vi "STM_Server.vi"() -> ()   [LabVIEW 2019, in "RemoteControl.STM.lvclass"]
uses:
  RemoteControl.STM.lvclass
  <vilib>/NI/STM/SubVIs/MetaDataElement.ctl
  <vilib>/NI/STM/TCP/Write Meta Data (TCP Ref).vi
  <vilib>/NI/STM/TCP/Get Connection Reference (TCP).vi
  <vilib>/NI/STM/TCP/Write Meta Data (TCP Clst).vi
  <vilib>/NI/STM/TCP/Read Message (TCP).vi
  <vilib>/NI/STM/TCP/Write Message (TCP).vi
  <vilib>/NI/STM/NI STM.lvlib
panel:
  out "counter 2":u32
  out "counter":u32
  in  "service name":string
  out "remote address":string
  out "command received":T1
  in  "Enum":T2(ring)
  out "data received":string
  in  "stop":bool
  out "error out":errorcluster
  # "SERVER  (INSTRUMENT)"
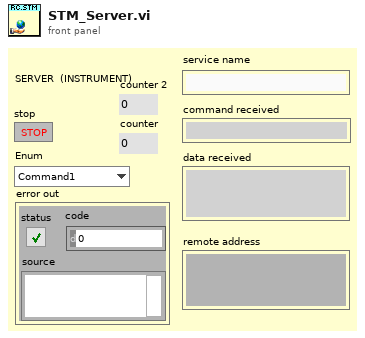
[diagram p1: front panel]
types:
  T1 = typedef "NI STM.lvlib/MetaDataElement.ctl" = string
  T2 = enum16{"Command1", "Command2", "Command3", "Command4", "HELP", "ACK", "CLOSE"}
  T3 = typedef "NI STM.lvlib/TCP Connection Info.ctl" = cluster{"connection ID":refnum<k5>, "meta data":T1[]}
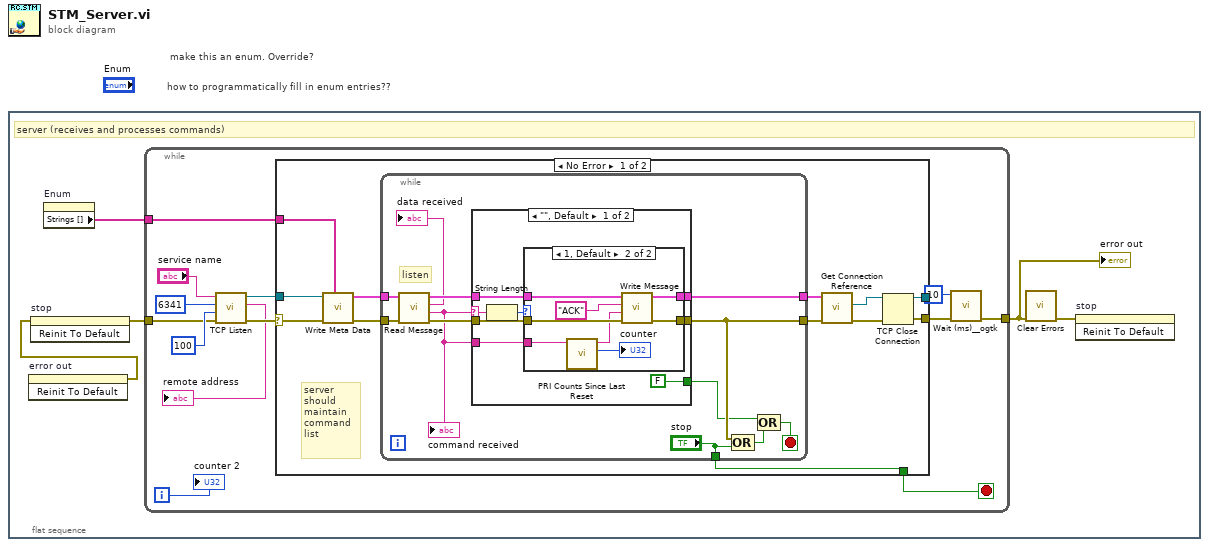
[diagram p0: block diagram]
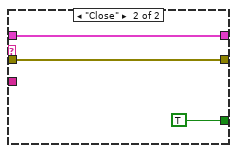
[diagram p3: hidden frame]
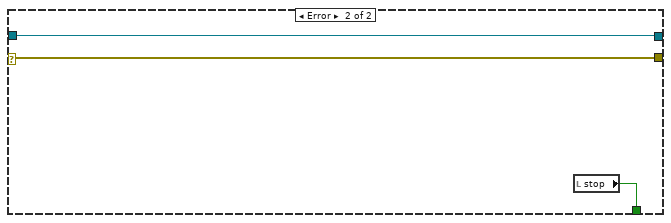
[diagram p4: hidden frame]
diagram:
  # "how to programmatically fill in enum entries??"
  # "make this an enum. Override?"
  n1 = flat-sequence {
    frame #0 {
      # "server (receives and processes commands)"
      n2 = invoke on="error out" class="Clust (strict)" method="Reinit To Default"() -> (error out=w1:errorcluster)  [unwired: 3 in, 2 out]
      n3 = invoke on="stop" class="Bool (strict)" method="Reinit To Default"(error in=w1) -> (error out=w5:errorcluster)  [unwired: 2 in, 2 out]
      n4 = property on="Enum" class="Enum (strict)"() -> ("Strings []"=w2:string[])  [unwired: 2 in, 2 out]
      n5 = while {
        tunnel: w5 -> [w13]
        tunnel: [w8] -> w3
        tunnel: w2 -> [w12]
        i -> [w6]
        stop <- w16 stop-if-true
        n6 = call <vilib>:"TCP Listen.vi"("error in (no error)"=w13, "timeout ms (wait forever: -1)"=100, "port"=u16 6341 ("remote port or service name"), "service name"="service name") -> ("error out"=w14:errorcluster, "remote address"=→"remote address":string, "connection ID"=w17:refnum<k5>)  [unwired: 3 in, 2 out]
        n7 = case shown="No Error" w14 {
          selector: w14 -> [w24 w64]
          tunnel: w17 -> [w23 w63]
          tunnel: [w26 w65] -> w16
          tunnel: [w25 w64] -> w9
          tunnel: w12 -> [w20 _]
          tunnel: [w19 w63] -> _
          frame No Error {
            # "server\nshould \nmaintain\ncommand\nlist"
            n8 = call-poly <vilib>:"Write Meta Data.vi"("meta data"=w20, "error in"=w24, "connection ID"=w23) -> ("error out"=w21:errorcluster, "connection info out"=w22:T3)  [unwired: 7 in]
            n9 = while {
              tunnel: w22 -> [w42]
              tunnel: w21 -> [w41]
              tunnel: [w37] -> w30
              tunnel: [w38] -> w29
              tunnel: ["stop"] -> w26
              stop <- w35 stop-if-true
              # "listen"
              n10 = call-poly <vilib>:"Read Message.vi"("error in"=w41, "connection info in"=w42) -> ("error out"=w40:errorcluster, "name"=w31:T1, "data string"=→"data received":string, "connection info out"=w39:T3)  [unwired: 4 in, 2 out]
              "command received" <- w31
              n11 = case shown="\"\", Default" w31 {
                selector: w31 -> [w45 _]
                tunnel: w40 -> [w47 w62]
                tunnel: w39 -> [w49 w61]
                tunnel: [w46 w62] -> w37
                tunnel: [w48 w61] -> w38
                tunnel: [FALSE ("value") TRUE ("value")] -> w34
                tunnel: w31 -> [w43 _]
                frame "", Default {
                  n12 = String Length(string=w45) -> (length=w44:i32)
                  n13 = case shown="1, Default" w44 {
                    tunnel: w49 -> [w51 w58]
                    tunnel: [w51 w57] -> w48
                    tunnel: w47 -> [w52 w56]
                    tunnel: [w52 w55] -> w46
                    tunnel: w43 -> [_ w54]
                    frame 0 {
                    }
                    frame 1, Default {
                      n14 = call "PRI Counts Since Last Reset.vi"() -> ("counter"=→"counter":u32)  [unwired: 6 in, 1 out]
                      n15 = call-poly <vilib>:"Write Message.vi"("error in"=w56, "data"=w54, "name"="ACK", "connection info in"=w58) -> ("error out"=w55:errorcluster, "connection info out"=w57:T3)  [unwired: 6 in]
                    }
                  }
                }
                frame "Close" {
                }
              }
              n16 = Compound Arithmetic op=OR(w37, "stop") -> (w36:bool)
              n17 = Compound Arithmetic op=OR(w34, w36) -> (w35:bool)
            }
            n18 = call-poly <vilib>:"Get Connection Reference.vi"("error in"=w30, "connection info in"=w29) -> ("error out"=w28:errorcluster, "connection ID out"=w27:refnum<k5>)  [unwired: 7 in, 1 out]
            n19 = TCP Close Connection(connection ID=w27, error in (no error)=w28) -> (connection ID out=w19:refnum<k5>, error out=w25:errorcluster)  [unwired: 1 in]
          }
          frame Error {
            n20 = local read "stop"() -> (w65:bool)
          }
        }
        n21 = call <userlib>:"Wait (ms)__ogtk.vi"("error in (no error)"=w9, "milliseconds to wait"=u32 10) -> ("error out"=w8:errorcluster)  [unwired: 8 in, 1 out]
        "counter 2" <- w6
      }
      "error out" <- w3
      n22 = call <vilib>:"Clear Errors.vi"("error in (no error)"=w3) -> ("error out"=w4:errorcluster)  [unwired: 5 in, 1 out]
      n23 = invoke on="stop" class="Bool (strict)" method="Reinit To Default"(error in=w4) -> ()  [unwired: 2 in, 3 out]
    }
  }
